vi "Configure Response - Wait (sec).vi"(8 "error in (no error)":errorcluster, 10 "settings":T1 {"Channel Refnum" format="%.0x"; "Linked Channels"."Channel Refnum" format="%.0x"}, 11 "reponse refnum in":T3 format="%.0x") -> (0 "error out":errorcluster, 3 "response refnum out":T3 format="%.0x")   [LabVIEW 2018, in "Instrument Addon Scripting API.lvlib"]
doc: "Configures the Response used as an input with the provided settings.\n\nIf you want to use \"Linked Channels\" with the \"Response Format\" string, make sure that the Channel Refnums used in the \"Linked Channels\" parameter already exist before calling this SubVI.\n\nNotes: \n- This VI will throw an error if the \"Response Format\" string contains duplicate variable names\n- This VI will throw an error if the number of variables in the \"Response Format\" string is different from the number of linked channels \n- This VI will throw an error if the variable names in the \"Response Format\" string does not correspond to the variable names used in the \"Linked Channels\" parameter."
uses:
  Instrument Addon Scripting API.lvlib
  <vilib>/NI Veristand/Custom Device API/Custom Device Item Ref.ctl
  TypeDefs/Wait Response Settings.ctl
  TypeDefs/Linked Channel.ctl
  Addon/Addon Shared/Types/FG Control.ctl
  Addon/Addon Shared/Types/Response Parameters.ctl
  Addon/Addon Shared/Types/Linked Channel Cluster.ctl
  Addon/Addon Shared/Types/Response Wait Type.ctl
  Addon/Addon Shared/SubVIs/Constants.vi
  <vilib>/NI Veristand/Custom Device API/NI VeriStand - Get Item Property.vi
  <vilib>/NI Veristand/Custom Device API/Get Item Property (String).vi
  <vilib>/NI Veristand/Custom Device API/Get Item Property (String Array).vi
  <vilib>/NI Veristand/Custom Device API/Get Item Property (Double).vi
  <vilib>/NI Veristand/Custom Device API/Get Item Property (U32).vi
  <vilib>/NI Veristand/Custom Device API/Get Item Property (Boolean).vi
  <vilib>/NI Veristand/Custom Device API/NI VeriStand - Set Item Property.vi
  <vilib>/NI Veristand/Custom Device API/Set Item Property (String).vi
  <vilib>/NI Veristand/Custom Device API/Set Item Property (String Array).vi
  <vilib>/NI Veristand/Custom Device API/Set Item Property (Double).vi
  <vilib>/NI Veristand/Custom Device API/Set Item Property (U32).vi
  <vilib>/NI Veristand/Custom Device API/Set Item Property (Boolean).vi
  Addon/Addon Shared/Instrument Addon Shared.lvlib
  <vilib>/NI Veristand/Custom Device API/Custom Device API.lvlib
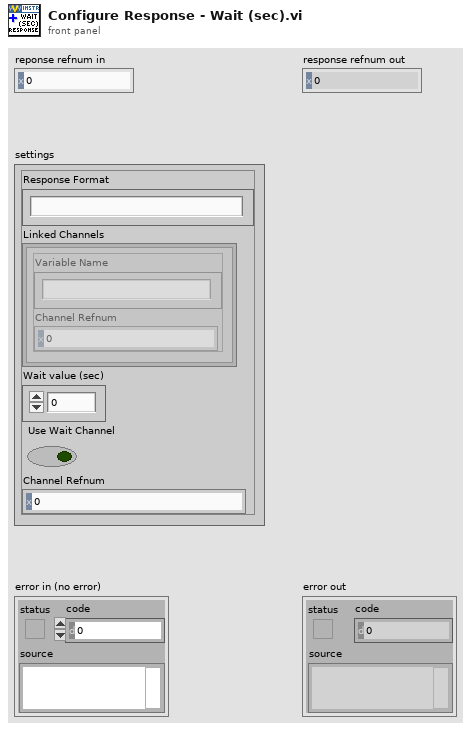
[diagram p1: front panel]
types:
  T1 = typedef "Instrument Addon Scripting API.lvlib/Wait Response Settings.ctl" = cluster{"Response Format":string, "Linked Channels":T2[], "Wait value (sec)":dbl, "Use Wait Channel":bool, "Channel Refnum":T3}
  T2 = typedef "Instrument Addon Scripting API.lvlib/Linked Channel.ctl" = cluster{"Variable Name":string, "Channel Refnum":T3}
  T3 = typedef "Custom Device API.lvlib/Custom Device Item Ref.ctl" = u64
  T4 = typedef "Instrument Addon Shared.lvlib/Response Wait Type.ctl" = enum16{"Byte Count", "Wait sec"}
  T5 = typedef "Instrument Addon Shared.lvlib/Response Parameters.ctl" = cluster{"Response":string, "Linked Channels":T6[], "Type Value":dbl, "Wait Type":T4, "Use Channel":bool, "Channel Path":string}
  T6 = typedef "Instrument Addon Shared.lvlib/Linked Channel Cluster.ctl" = cluster{"Variable Name":string, "GUID":string}
  T7 = typedef "Instrument Addon Shared.lvlib/FG Control.ctl" = enum16{"Get", "Set"}
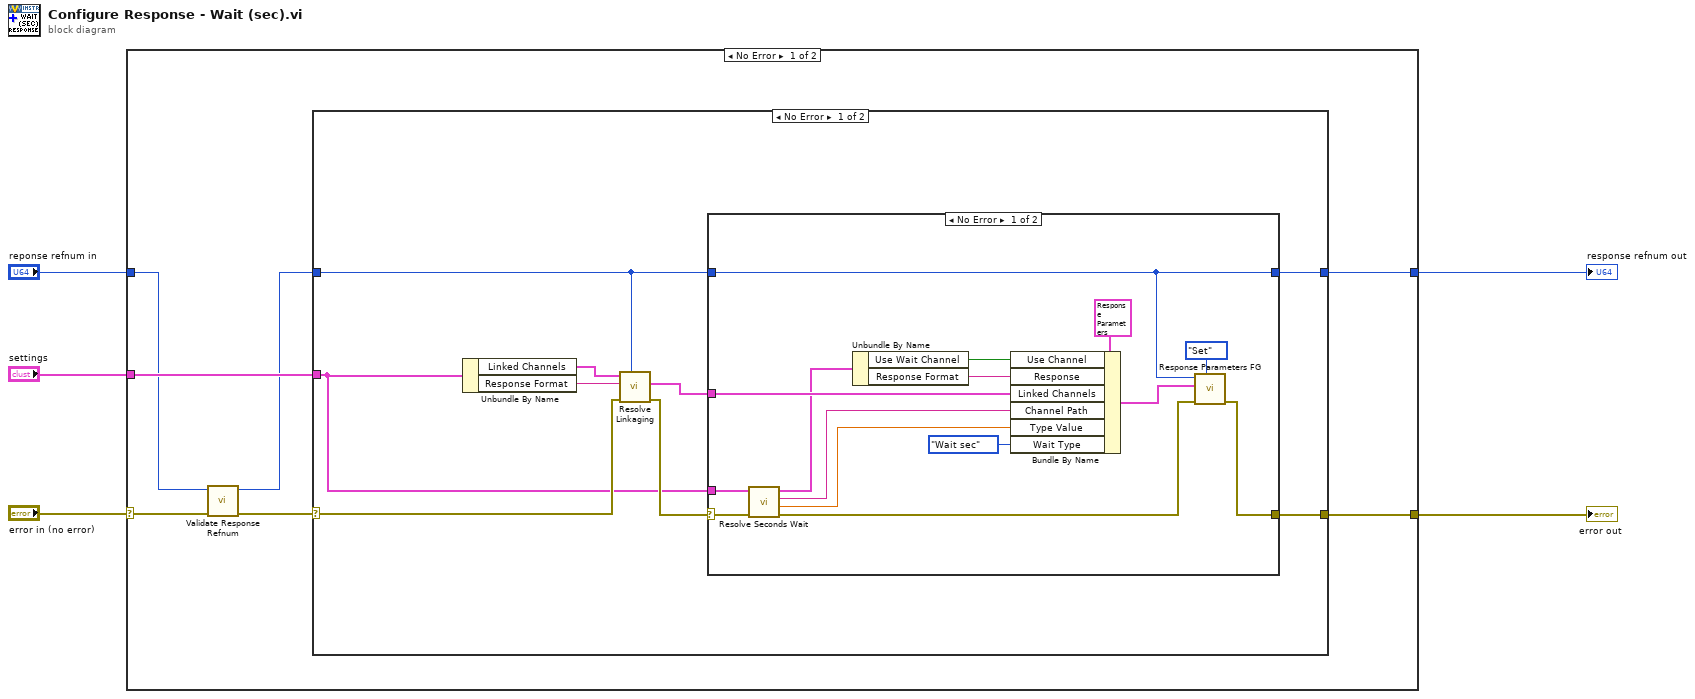
[diagram p0: block diagram]
diagram:
  n1 = case shown="No Error" "error in (no error)" {
    selector: "error in (no error)" -> [w7 w41]
    tunnel: "reponse refnum in" -> [w9 w42]
    tunnel: "settings" -> [w12 _]
    tunnel: [w11 w42] -> w3
    tunnel: [w10 w41] -> w2
    frame No Error {
      n2 = call "Validate Response Refnum.vi"("error in (no error)"=w7, "response refnum in"=w9) -> ("error out"=w6:errorcluster, "response refnum out"=w8:u64)  [unwired: 8 in]
      n3 = case shown="No Error" w6 {
        selector: w6 -> [w15 w39]
        tunnel: w12 -> [w13 _]
        tunnel: [w21 w40] -> w11
        tunnel: [w20 w39] -> w10
        tunnel: w8 -> [w14 w40]
        frame No Error {
          n4 = Unbundle By Name(w13) -> ("Linked Channels"=w16:T2[], "Response Format"=w17:string)
          n5 = call "Resolve Linkaging.vi"("Command/Response Refnum in"=w14, "error in (no error)"=w15, "Command/Response Format"=w17, "Linked Channels"=w16) -> ("error out"=w19:errorcluster, "Linked Channels out"=w18:T6[])  [unwired: 6 in]
          n6 = case shown="No Error" w19 {
            selector: w19 -> [w28 w37]
            tunnel: w18 -> [w32 _]
            tunnel: [w31 w37] -> w20
            tunnel: w14 -> [w22 w38]
            tunnel: [w22 w38] -> w21
            tunnel: w13 -> [w24 _]
            frame No Error {
              n7 = call "Resolve Seconds Wait.vi"("error in (no error)"=w28, "Settings in"=w24) -> ("error out"=w26:errorcluster, "Wait value (sec)"=w23:dbl, "Channel Path"=w25:string, "Settings out"=w27:T1)  [unwired: 6 in]
              n8 = Unbundle By Name(w27) -> ("Use Wait Channel"=w29:bool, "Response Format"=w34:string)
              n9 = Bundle By Name(cluster=T5 {"Response"="", "Linked Channels"=[], "Type Value"=1.0, "Wait Type"=enum."Wait sec", "Use Channel"=FALSE, "Channel Path"=""} ("Reponse Parameters"), "Use Channel"=w29, "Response"=w34, "Linked Channels"=w32, "Channel Path"=w25, "Type Value"=w23, "Wait Type"=Response_Wait_Type."Wait sec") -> (w33:T5)
              n10 = call "Response Parameters FG.vi"("Action"=FG_Control."Set", "error in (no error)"=w26, "Reponse Parameters"=w33, "Item Ref in"=w22) -> ("error out"=w31:errorcluster)  [unwired: 5 in, 2 out]
            }
            frame Error {
            }
          }
        }
        frame Error {
        }
      }
    }
    frame Error {
    }
  }
  "error out" <- w2
  "response refnum out" <- w3
